vi "Cyborg_Position_Control_Spark.vi"(0 "MotorControlDevRef":T2={"DeviceStatus"={"status"=FALSE, "code"=0, "source"=""}, "Type"=enum."PWM", "PWM"={"PWM Channel"=enum."PWM 1", "DeadBand"={"Name"="", "maxPositivePwm"=0, "minPositivePwm"=0, "centerPwm"=0, "maxNegativePwm"=0, "minNegativePwm"=0, "angularRange"=0}}, "CAN"={"Device Number"=0, "SetOutput VI Ref"=variant(enum8{"Percent VBus", "Current", "Speed", "Position", "Voltage"} enum."Percent VBus"), "GetOutput VI Ref"=variant(refnum<k1> refnum), "Enable VI Ref"=variant(dbl 12.0), "Disable VI Ref"=variant(enum8{"Percent VBus", "Speed", "Position", "Slave", "Unchanged / Invalid", "Voltage Compensation", "Current", "Motion Profile"} enum."Percent VBus"), "Data"=variant}, "Invert"=FALSE, "DIO PWM"={"PWM \"Enable\" Channel"=enum."Invalid", "DIOChannel"=enum."Invalid", "PWM Rate"=0.0}}, 2 "Upper":bool, 3 "Lower":bool, 5 "Jog Input":dbl, 6 "Lower":dbl, 7 "Higher":dbl, 10 "Drive Feedback":bool) -> ()   [LabVIEW 2020]
uses:
  <vilib>/Rock Robotics/WPI/MotorControl/WPI_MotorControlDeviceRef.ctl
  <vilib>/Rock Robotics/WPI/MotorControl/WPI_MotorControlType.ctl
  <vilib>/Rock Robotics/SystemInterfaces/DIO/FPGA_DIOPWMChannel.ctl
  <vilib>/Rock Robotics/WPI/PWM/WPI_PWMDeadband.ctl
  <vilib>/Rock Robotics/SystemInterfaces/DIO/FPGA_DIOChannel.ctl
  <vilib>/Rock Robotics/WPI/ThirdParty/REV Robotics/REVLib/Typedef/Spark MAX Control Type.ctl
  <vilib>/Rock Robotics/Network Tables/NT Write Number.vi
panel:
  in  "PID Constants":T1={"P Gain"=1.0, "I Gain"=0.0, "D Gain"=0.0, "F Gain"=0.0, "I Zone"=0.0, "Min Output"=-1.0, "Max Output"=1.0}
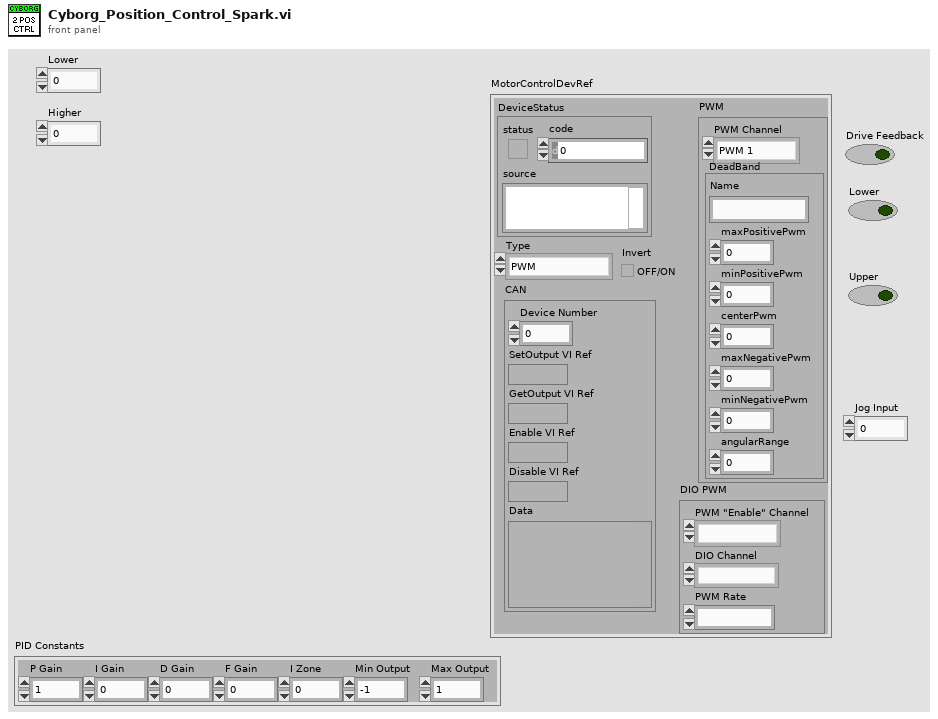
[diagram p1: front panel]
types:
  T1 = cluster{"P Gain":dbl, "I Gain":dbl, "D Gain":dbl, "F Gain":dbl, "I Zone":dbl, "Min Output":dbl, "Max Output":dbl}
  T2 = typedef "WPI_MotorControlDeviceRef.ctl" = cluster{"DeviceStatus":errorcluster, "Type":T3, "PWM":cluster{"PWM Channel":T4, "DeadBand":T5}, "CAN":cluster{"Device Number":u8, "SetOutput VI Ref":variant, "GetOutput VI Ref":variant, "Enable VI Ref":variant, "Disable VI Ref":variant, "Data":variant}, "Invert":bool, "DIO PWM":cluster{"PWM \"Enable\" Channel":T4, "DIOChannel":T6, "PWM Rate":dbl}}
  T3 = typedef "WPI_MotorControlType.ctl" = enum16{"PWM", "CAN", "DIO PWM"}
  T4 = typedef "FPGA_DIOPWMChannel.ctl" = enum8{"PWM 0", "PWM 1", "PWM 2", "PWM 3", "PWM 4", "PWM 5", "PWM 6", "PWM 7", "PWM 8", "PWM 9", "PWM MXP 0", "PWM MXP 1", "PWM MXP 2", "PWM MXP 3", "PWM MXP 4", "PWM MXP 5", "PWM MXP 6", "PWM MXP 7", "PWM MXP 8", "PWM MXP 9", "Invalid"}
  T5 = typedef "WPI_PWMDeadband.ctl" = cluster{"Name":string, "maxPositivePwm":i32, "minPositivePwm":i32, "centerPwm":i32, "maxNegativePwm":i32, "minNegativePwm":i32, "angularRange":u16}
  T6 = typedef "FPGA_DIOChannel.ctl" = enum8{"DIO 0", "DIO 1", "DIO 2", "DIO 3", "DIO 4", "DIO 5", "DIO 6", "DIO 7", "DIO 8", "DIO 9", "DIO MXP 0", "DIO MXP 1", "DIO MXP 2", "DIO MXP 3", "DIO MXP 4", "DIO MXP 5", "DIO MXP 6", "DIO MXP 7", "DIO MXP 8", "DIO MXP 9", "DIO MXP 10", "DIO MXP 11", "DIO MXP 12", "DIO MXP 13", "DIO MXP 14", "DIO MXP 15", "SPI Port CS1", "SPI Port CS2", "SPI Port CS3", "SPI Port MISO", "SPI Port MOSI", "Invalid"}
  T7 = typedef "Spark MAX Control Type.ctl" = enum16{"Percent VBus", "Voltage", "Velocity", "Position", "Smart Motion", "Current", "Smart Velocity"}
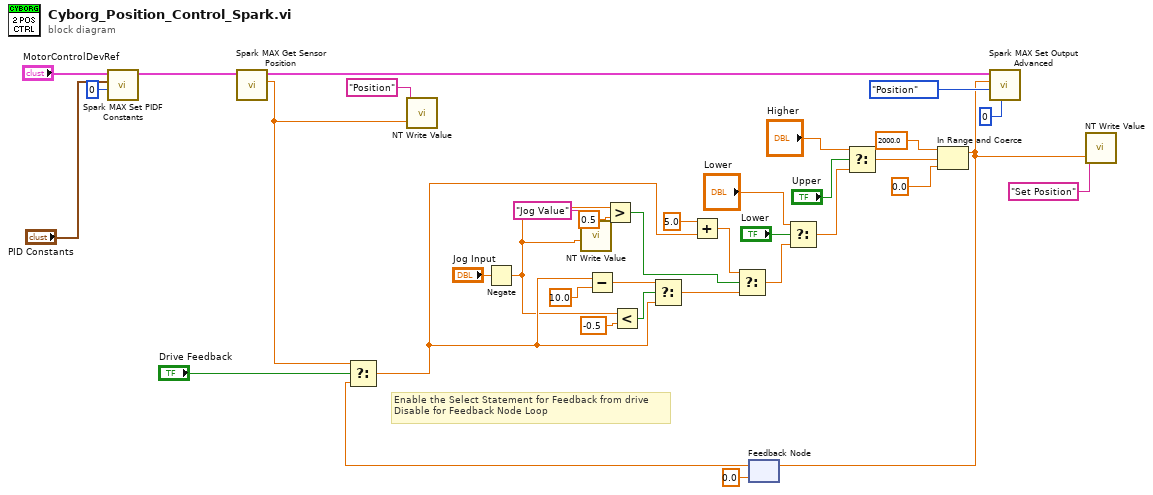
[diagram p0: block diagram]
diagram:
  # "Enable the Select Statement for Feedback from drive\nDisable for Feedback Node Loop"
  n1 = call <vilib>:"Spark MAX Set PIDF Constants.vi"("PIDF Slot"=0, "PID Constants"="PID Constants", "MotorControlDeviceRef"="MotorControlDevRef") -> ("MotorControlDeviceRef"=w12:T2)  [unwired: 7 in, 1 out]
  n2 = call <vilib>:"Spark MAX Get Sensor Position.vi"("MotorControlDevRef in"=w12) -> ("Sensor Position"=w8:dbl, "MotorControlDevRef out"=w22:T2)  [unwired: 7 in, 2 out]
  n3 = call-poly <vilib>:"NT Write Value.vi"("timestamp"=w8, "name"="Position") -> ()  [unwired: 9 in, 1 out]
  n4 = Negate(x="Jog Input") -> (-x=w1:dbl)
  n5 = call-poly <vilib>:"NT Write Value.vi"("value"=w1, "name"="Jog Value") -> ()  [unwired: 9 in, 1 out]
  n6 = Greater?(x=w1, y=0.5) -> (0:w29:bool)
  n7 = Less?(x=w1, y=-0.5) -> (x < y?=w30:bool)
  n8 = feedback #1(0.0 ("upper limit")) -> (w18:dbl)
  n9 = Select(t=w8, s="Drive Feedback", f=w18) -> (s? t:f=w19:dbl)
  n10 = Subtract(x=w19, y=10.0 ("Jog Counts")) -> (x-y=w23:dbl)
  n11 = Select(t=w23, s=w30, f=w19) -> (s? t:f=w25:dbl)
  n12 = Add(x=5.0 ("Jog Counts"), y=w19) -> (x+y=w26:dbl)
  n13 = Select(t=w26, s=w29, f=w25) -> (s? t:f=w33:dbl)
  n14 = Select(t="Lower", s="Lower", f=w33) -> (s? t:f=w36:dbl)
  n15 = Select(t="Higher", s="Upper", f=w36) -> (s? t:f=w15:dbl)
  n16 = In Range and Coerce(upper limit=2000.0, x=w15, lower limit=0.0) -> (coerced(x)=w7:dbl)  [unwired: 1 out]
  n17 = feedback-in #1(w7) -> ()
  n18 = call <vilib>:"Spark MAX Set Output Advanced.vi"("PIDF Slot (0)"=0, "Control Mode"=Spark_MAX_Control_Type."Position", "Setpoint"=w7, "MotorControlDevRef"=w22) -> ()  [unwired: 6 in, 2 out]
  n19 = call-poly <vilib>:"NT Write Value.vi"("timestamp"=w7, "name"="Set Position") -> ()  [unwired: 9 in, 1 out]
